vi "与工控机交互(子VI).vi"   [LabVIEW 2016, in "数据传输系统.lvlib"]
uses:
  <vilib>/ptbypt/NI_PtbyPt.lvlib
types:
  T1 = cluster{"setini":string, "sysini":string, "hechaini":string, "actualwrite":string, "actualread":string, "datasent":string, "反控命令信息队列":string, "反控与仪器交互":string}
  T2 = cluster{"[0]":bool, "[1]":bool, "[2]":bool, "[3]":bool, "[4]":bool}
  T3 = cluster{"[0]":bool, "[1]":bool, "[2]":bool, "[3]":bool, "[4]":bool, "[5]":bool}
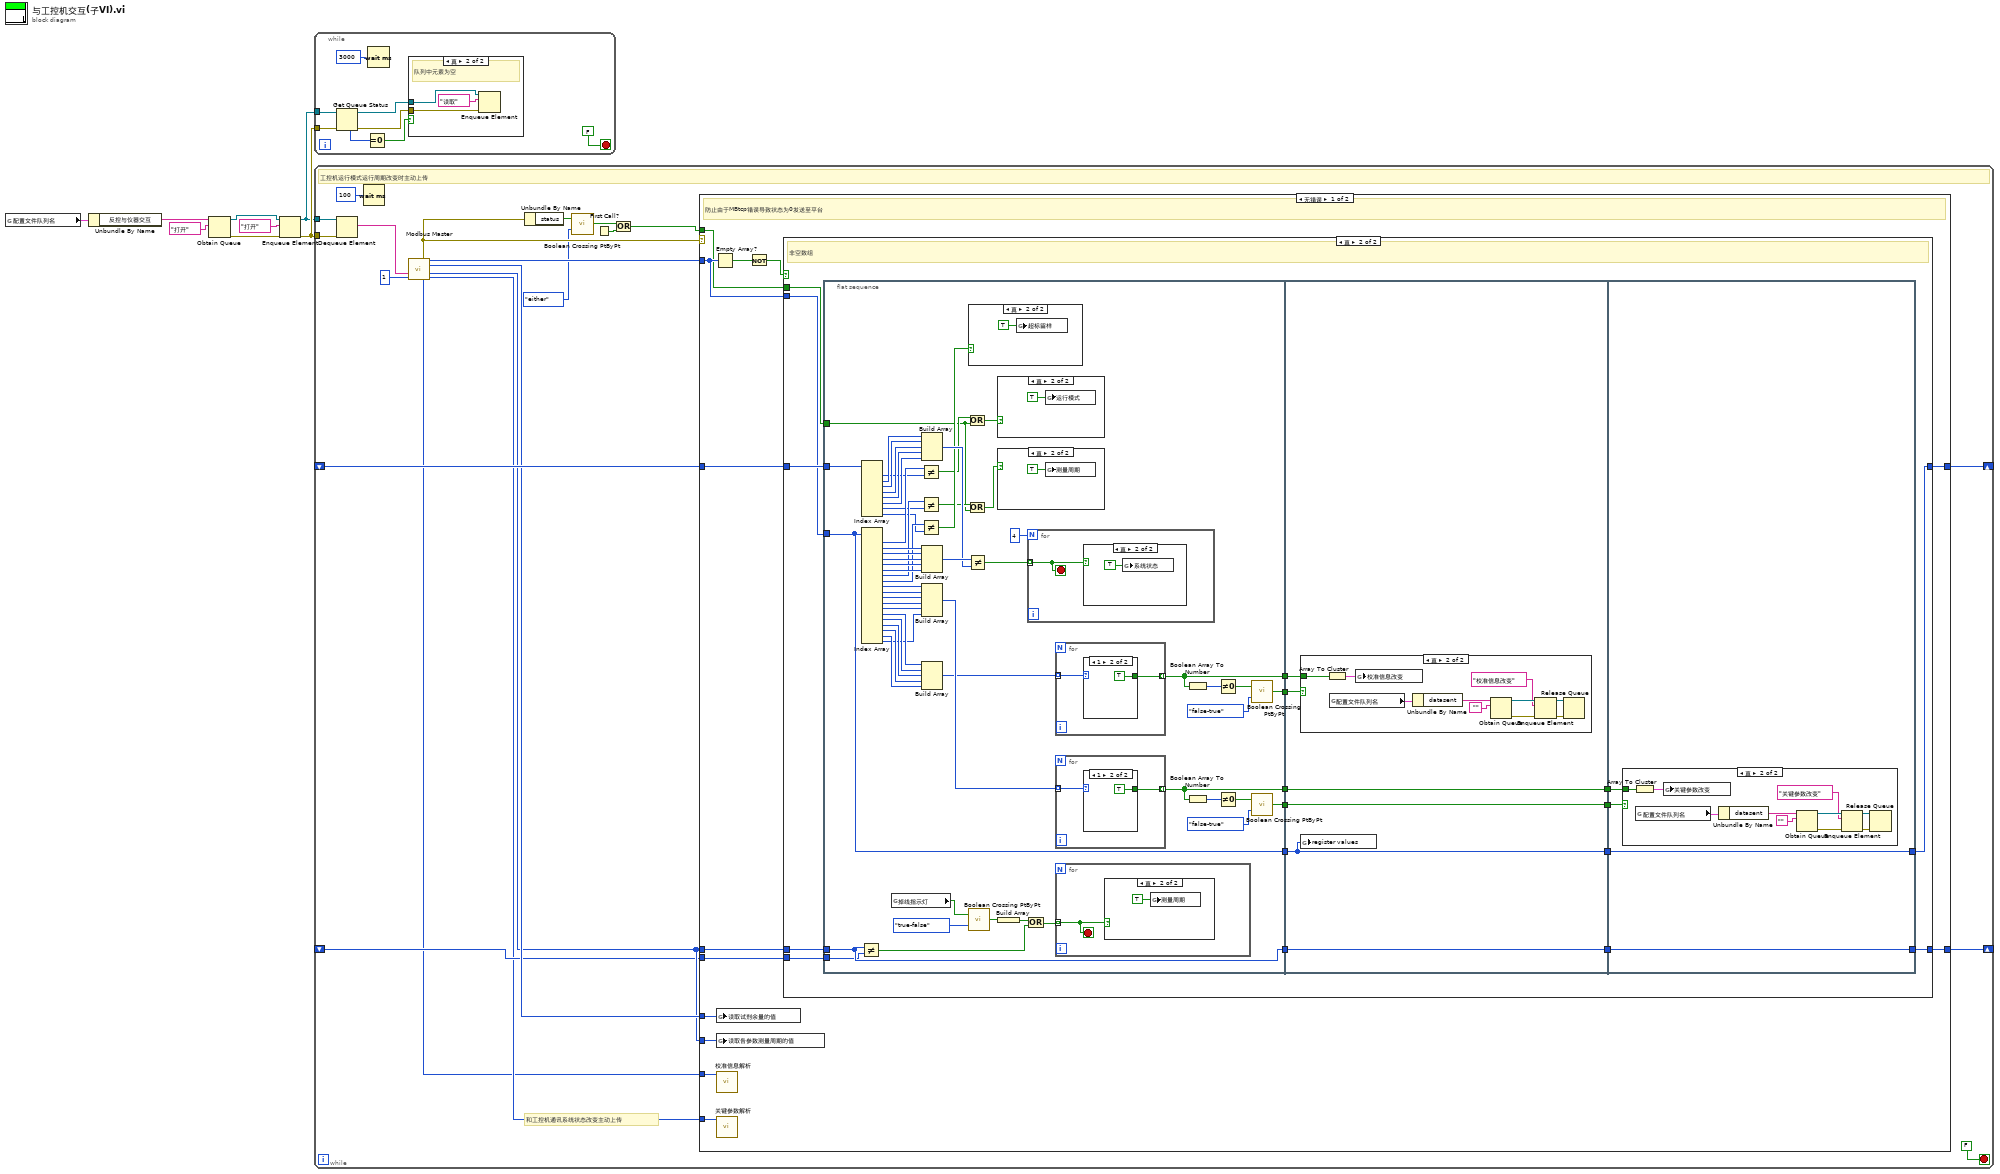
[diagram p0: block diagram]
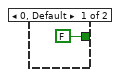
[diagram p4: hidden frame]
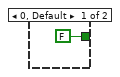
[diagram p5: hidden frame]
diagram:
  n1 = global read "断电保存全局.vi" "配置文件队列名"() -> (w2:T1)
  n2 = Unbundle By Name(w2) -> ("反控与仪器交互"=w1:string)
  n3 = Obtain Queue(name (unnamed)=w1, element data type="打开" ("读取写入选择")) -> (queue out=w4:refnum<queue>, error out=w5:errorcluster)  [unwired: 3 in, 1 out]
  n4 = Enqueue Element(queue=w4, element="打开" ("读取写入选择"), error in (no error)=w5) -> (queue out=w6:refnum<queue>, error out=w7:errorcluster)  [unwired: 1 in, 1 out]
  n5 = while {
    tunnel: w6 -> [w13]
    tunnel: w7 -> [w12]
    stop <- FALSE stop-if-true
    n6 = Get Queue Status(queue=w13, error in (no error)=w12) -> (queue out=w10:refnum<queue>, error out=w9:errorcluster, # elements in queue=w14:i32)  [unwired: 1 in, 5 out]
    n7 = Equal To 0?(x=w14) -> (x = 0?=w11:bool)
    n8 = Wait (ms)(milliseconds to wait=u32 3000 ("等待时间（毫秒）")) -> ()  [unwired: 1 out]
    n9 = case shown="真" w11 {
      tunnel: w10 -> [_ w18]
      tunnel: w9 -> [_ w17]
      frame False {
      }
      frame True {
        # "队列中元素为空"
        n10 = Enqueue Element(queue=w18, element="读取" ("读取写入选择"), error in (no error)=w17) -> ()  [unwired: 1 in, 3 out]
      }
    }
  }
  n11 = while {
    tunnel: w6 -> [w36]
    tunnel: w7 -> [w35]
    shift-right: [w32] -> _
    shift-left: _ -> [w33]
    shift-right: [w23] -> _
    shift-left: _ -> [w22]
    stop <- FALSE stop-if-true
    # "和工控机通讯系统状态改变主动上传"
    # "工控机运行模式运行周期改变时主动上传"
    n12 = Dequeue Element(queue=w36, error in (no error)=w35) -> (element=w34:string)  [unwired: 1 in, 3 out]
    n13 = Wait (ms)(milliseconds to wait=u32 100 ("等待时间（毫秒）")) -> ()  [unwired: 1 out]
    n14 = call "Modbus Master.vi"("读取写入选择"=w34, "Unit ID"=u8 1) -> ("error out"=w31:errorcluster, "仪器状态"=w38:u16[], "试剂余量"=w25:u16[], "各参数测量间隔"=w24:u16[], "校准点信息"=w20:u16[], "关键参数"=w21:u16[])  [unwired: 8 in]
    n15 = Unbundle By Name(w31) -> ("status"=w30:bool)
    n16 = call <vilib>:"Boolean Crossing PtByPt.vi"("direction"=enum16{"either", "false-true", "true-false"}."either", "input"=w30) -> ("crossing"=w28:bool)  [unwired: 1 in]
    n17 = First Call?() -> (First Call?: T/F=w27:bool)
    n18 = Or(x=w28, y=w27) -> (x .or. y?=w26:bool)
    n19 = case shown="无错误" w31 {
      tunnel: w38 -> [w51 _]
      tunnel: w33 -> [w53 w178]
      tunnel: [w52 w178] -> w32
      tunnel: w26 -> [w48 _]
      tunnel: w25 -> [w47 _]
      tunnel: w24 -> [w46 _]
      tunnel: w24 -> [w45 w177]
      tunnel: [w44 w177] -> w23
      tunnel: w22 -> [w43 _]
      tunnel: w21 -> [w42 _]
      tunnel: w20 -> [w41 _]
      frame No Error {
        # "防止由于MBtcp错误导致状态为0发送至平台"
        n20 = Empty Array?(array=w51) -> (empty?=w50:bool)
        n21 = global write "全局1.vi" "读取试剂余量的值"(w47) -> ()
        n22 = global write "全局1.vi" "读取各参数测量周期的值"(w46) -> ()
        n23 = call "校准信息解析.vi"("校准信息"=w41) -> ()  [unwired: 11 in]
        n24 = call "关键参数解析.vi"("关键参数"=w42) -> ()  [unwired: 11 in]
        n25 = Not(x=w50) -> (.not. x?=w49:bool)
        n26 = case shown="真" w49 {
          tunnel: w53 -> [w55 w71]
          tunnel: [w55 w70] -> w52
          tunnel: w51 -> [_ w69]
          tunnel: w48 -> [_ w68]
          tunnel: w45 -> [w54 w67]
          tunnel: [w54 w65] -> w44
          tunnel: w43 -> [_ w64]
          frame False {
          }
          frame True {
            # "非空数组"
            n27 = flat-sequence {
              tunnel: w69 -> [w115]
              tunnel: [w115] -> w72
              tunnel: w71 -> [w111]
              tunnel: w68 -> [w106]
              tunnel: w67 -> [w104]
              tunnel: [w104] -> w66
              tunnel: w64 -> [w103]
              tunnel: [w92] -> w63
              tunnel: [w81] -> w62
              tunnel: [w80] -> w61
              tunnel: [w79] -> w60
              tunnel: w72 -> [w152]
              tunnel: w66 -> [w151]
              tunnel: w63 -> [w147]
              tunnel: w62 -> [w150]
              tunnel: w61 -> [w149]
              tunnel: w60 -> [w148]
              tunnel: [w152] -> w59
              tunnel: [w151] -> w58
              tunnel: [w148] -> w57
              tunnel: [w147] -> w56
              tunnel: [w165] -> w65
              tunnel: [w166] -> w70
              tunnel: w59 -> [w166]
              tunnel: w58 -> [w165]
              tunnel: w57 -> [w164]
              tunnel: w56 -> [w163]
              frame #0 {
                n28 = Not Equal?(x=w104, y=w103) -> (x != y?=w102:bool[])
                n29 = Index Array(array=w111) -> (element #1=w118:u16, element #2=w126:u16, element #3=w125:u16, element #4=w124:u16, element #5=w123:u16, element #6=w122:u16, element #7=w116:u16, element #8=w113:u16)  [unwired: 8 in]
                n30 = Index Array(array=w115) -> (element #1=w119:u16, element #2=w131:u16, element #3=w130:u16, element #4=w129:u16, element #5=w128:u16, element #6=w127:u16, element #7=w117:u16, element #8=w114:u16, element #9=w100:u16, element #10=w99:u16, element #11=w98:u16, element #12=w97:u16, element #13=w96:u16, element #14=w90:u16, element #15=w89:u16, element #16=w88:u16, element #17=w87:u16, element #18=w86:u16, element #19=w73:u16)  [unwired: 19 in]
                n31 = global read "全局 数据发送重叠.vi" "掉线指示灯"() -> (w77:bool)
                n32 = Not Equal?(x=w119, y=w118) -> (x != y?=w109:bool)
                n33 = Not Equal?(x=w117, y=w116) -> (x != y?=w107:bool)
                n34 = Not Equal?(x=w114, y=w113) -> (x != y?=w112:bool)
                n35 = Build Array(w126, w125, w124, w123, w122) -> (w120:u16[])
                n36 = Build Array(w131, w130, w129, w128, w127) -> (w121:u16[])
                n37 = Build Array(w100, w99, w98, w97, w96, w73) -> (w95:u16[])
                n38 = Build Array(w90, w89, w88, w87, w86) -> (w82:u16[])
                n39 = Or(x=w109, y=w106) -> (x .or. y?=w108:bool)
                n40 = Or(x=w107, y=w106) -> (x .or. y?=w105:bool)
                n41 = Not Equal?(x=w121, y=w120) -> (x != y?=w110:bool[])
                n42 = case shown="真" w112 {
                  frame False {
                  }
                  frame True {
                    n43 = global write "全局1.vi" "超标留样"(TRUE ("系统状态改变")) -> ()
                  }
                }
                n44 = call <vilib>:"Boolean Crossing PtByPt.vi"("direction"=enum16{"either", "false-true", "true-false"}."true-false", "input"=w77) -> ("crossing"=w75:bool)  [unwired: 1 in]
                n45 = case shown="真" w108 {
                  frame False {
                  }
                  frame True {
                    n46 = global write "全局1.vi" "运行模式"(TRUE) -> ()
                  }
                }
                n47 = case shown="真" w105 {
                  frame False {
                  }
                  frame True {
                    n48 = global write "全局1.vi" "测量周期"(TRUE ("系统状态改变")) -> ()
                  }
                }
                n49 = Build Array(w75) -> (w74:bool[])
                n50 = Or(x=w74, y=w102) -> (x .or. y?=w78:bool[])
                n51 = for {
                  N: 4 -> [_]
                  tunnel: w110 -> [w142] mode=indexing
                  stop <- w142 stop-if-true
                  n52 = case shown="真" w142 {
                    frame False {
                    }
                    frame True {
                      n53 = global write "全局1.vi" "系统状态"(TRUE ("系统状态改变")) -> ()
                    }
                  }
                }
                n54 = for {
                  tunnel: w82 -> [w133] mode=indexing
                  tunnel: [w132] -> w80 mode=indexing
                  n55 = case shown="1" w133 {
                    tunnel: [FALSE TRUE] -> w132
                    frame 0, Default {
                    }
                    frame 1 {
                    }
                  }
                }
                n56 = for {
                  tunnel: w95 -> [w137] mode=indexing
                  tunnel: [w136] -> w79 mode=indexing
                  n57 = case shown="1" w137 {
                    tunnel: [FALSE TRUE] -> w136
                    frame 0, Default {
                    }
                    frame 1 {
                    }
                  }
                }
                n58 = for {
                  tunnel: w78 -> [w140] mode=indexing
                  stop <- w140 stop-if-true
                  n59 = case shown="真" w140 {
                    frame False {
                    }
                    frame True {
                      n60 = global write "全局1.vi" "测量周期"(TRUE ("系统状态改变")) -> ()
                    }
                  }
                }
                n61 = Boolean Array To Number(Boolean array=w80) -> (number=w83:u32)
                n62 = Boolean Array To Number(Boolean array=w79) -> (number=w94:u32)
                n63 = Not Equal To 0?(x=w83) -> (x != 0?=w84:bool)
                n64 = Not Equal To 0?(x=w94) -> (x != 0?=w93:bool)
                n65 = call <vilib>:"Boolean Crossing PtByPt.vi"("direction"=enum16{"either", "false-true", "true-false"}."false-true", "input"=w84) -> ("crossing"=w81:bool)  [unwired: 1 in]
                n66 = call <vilib>:"Boolean Crossing PtByPt.vi"("direction"=enum16{"either", "false-true", "true-false"}."false-true", "input"=w93) -> ("crossing"=w92:bool)  [unwired: 1 in]
              }
              frame #1 {
                n67 = case shown="真" w150 {
                  tunnel: w149 -> [_ w153]
                  frame False {
                  }
                  frame True {
                    n68 = Array To Cluster(array=w153) -> (cluster=w154:T2)
                    n69 = global read "断电保存全局.vi" "配置文件队列名"() -> (w162:T1)
                    n70 = global write "全局1.vi" "校准信息改变"(w154) -> ()
                    n71 = Unbundle By Name(w162) -> ("datasent"=w161:string)
                    n72 = Obtain Queue(name (unnamed)=w161, element data type="") -> (queue out=w159:refnum<queue>, error out=w157:errorcluster)  [unwired: 3 in, 1 out]
                    n73 = Enqueue Element(queue=w159, element="校准信息改变" ("元素"), error in (no error)=w157) -> (queue out=w156:refnum<queue>, error out=w155:errorcluster)  [unwired: 1 in, 1 out]
                    n74 = Release Queue(queue=w156, error in (no error)=w155) -> ()  [unwired: 1 in, 3 out]
                  }
                }
                n75 = global write "全局1.vi" "register values"(w152) -> ()
              }
              frame #2 {
                n76 = case shown="真" w163 {
                  tunnel: w164 -> [_ w167]
                  frame False {
                  }
                  frame True {
                    n77 = Array To Cluster(array=w167) -> (cluster=w168:T3)
                    n78 = global read "断电保存全局.vi" "配置文件队列名"() -> (w176:T1)
                    n79 = global write "全局1.vi" "关键参数改变"(w168) -> ()
                    n80 = Unbundle By Name(w176) -> ("datasent"=w175:string)
                    n81 = Obtain Queue(name (unnamed)=w175, element data type="") -> (queue out=w173:refnum<queue>, error out=w171:errorcluster)  [unwired: 3 in, 1 out]
                    n82 = Enqueue Element(queue=w173, element="关键参数改变" ("元素"), error in (no error)=w171) -> (queue out=w170:refnum<queue>, error out=w169:errorcluster)  [unwired: 1 in, 1 out]
                    n83 = Release Queue(queue=w170, error in (no error)=w169) -> ()  [unwired: 1 in, 3 out]
                  }
                }
              }
            }
          }
        }
      }
      frame Error {
      }
    }
  }
